vi "Motors Modules Test.vi"(0 "All":T2={"I 1"=TRUE, "I 2"=FALSE, "I 3"=FALSE, "I 4"=TRUE}) -> ()   [LabVIEW 2015]
uses:
  <vilib>/FPGAPlugInAG/myRIO-1900/niLvFpga_Open_myRIO-1900.vi
  <vilib>/rvi/interface/common/dynamic/niFpgaDynamicAddResources.vi
  <vilib>/FPGAPlugInAG/Dynamic/niLvFpga_Run_Dynamic.vi
  <vilib>/FPGAPlugInAG/Dynamic/niLvFpga_Close_Dynamic.vi
  <vilib>/rvi/interface/nirviOpenFPGA/nirviOpenFPGA.xnode
  FPGA Bitfiles/PDMSMain_FPGATarget-Wi-Fi_Express2_Jo8xc+hAvHc.lvbitx
  FPGA/Express.vi
  <vilib>/rvi/interface/nirviMethod/nirviMethod.xnode
  <vilib>/rvi/interface/nirviCloseFPGA/nirviCloseFPGA.xnode
panel:
  in  "Speed":T1
  out "Error Out":errorcluster={"status"=FALSE, "code"=63186, "source"="niLvFpga_Open_myRIO-1900.vi"}
  in  "Error In":errorcluster
  in  "Stop Button":bool
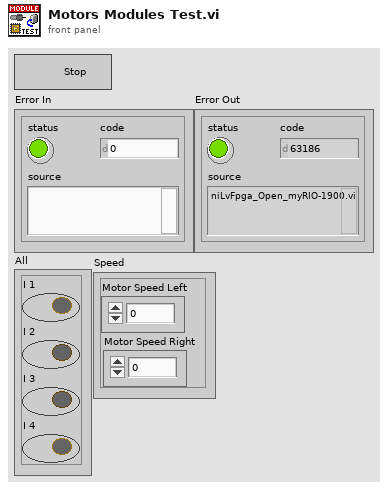
[diagram p1: front panel]
types:
  T1 = cluster{"Motor Speed Left":i16, "Motor Speed Right":i16}
  T2 = cluster{"I 1":bool, "I 2":bool, "I 3":bool, "I 4":bool}
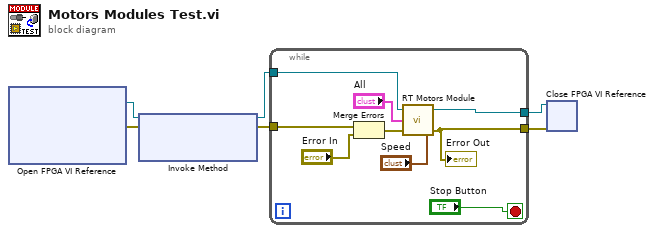
[diagram p0: block diagram]
diagram:
  n1 = xnode "Open FPGA VI Reference"() -> ("FPGA VI Reference Out"=w6:refnum<k20>, "error out"=w5:errorcluster)  [unwired: 2 in]
  n2 = xnode "Invoke Method"("FPGA VI Reference In"=w6, "error in"=w5) -> ("FPGA VI Reference Out"=w3:refnum<k20>, "error out"=w4:errorcluster)  [unwired: 1 in]
  n3 = while {
    tunnel: [w11] -> w1
    tunnel: [w10] -> w2
    tunnel: w4 -> [w9]
    tunnel: w3 -> [w8]
    stop <- "Stop Button" stop-if-true
    n4 = Merge Errors(w9, "Error In") -> (w13:errorcluster)
    n5 = call "RT Motors Module.vi"("Speed"="Speed", "Error In"=w13, "All"="All", "FPGA VI Reference In"=w8) -> ("Error Out"=w11:errorcluster, "FPGA VI Reference Out"=w10:refnum<k20>)
    "Error Out" <- w11
  }
  n6 = xnode "Close FPGA VI Reference"("FPGA VI Reference In"=w2, "error in"=w1) -> ()  [unwired: 1 out]
